vi "Set 1D Array String.vi"(5 "use temporary file? (F)":bool, 8 "error in":errorcluster, 9 "value":string[](array[string]), 10 "variable name":string, 11 "GOLPI ref. in":T1={"pipe handle"={"lv_proc.dll file path"=path "", "process instance handle"=[], "debug mode"=FALSE, "debug data"=[]}, "fast read timeout [ms]"=500, "fast read settle time [ms]"=10, "fast read to multiple [ms]"=1, "max elements per input line"=100, "slow read timeout [ms]"=5000, "stdin double format specifier"="%_16e", "max elements per stdout output column"=100, "console mode bitstream"=FALSE, "bitstream first read timeout [ms]"=1000, "bitstream read timeout [ms]"=50, "struct transfer possible"=FALSE, "matlab mode"=FALSE, "var pipe write timeout [ms]"=5000, "variable pipe mode"=FALSE, "variable pipe buffer size [Bytes]"=10000000, "variable pipe block size [Bytes]"=1000000} {"variable pipe block size [Bytes]" format="%.0p"; "variable pipe buffer size [Bytes]" format="%.0p"}) -> (0 "error out":errorcluster, 3 "GOLPI ref. out":T1={"pipe handle"={"lv_proc.dll file path"=path "", "process instance handle"=[], "debug mode"=FALSE, "debug data"=[]}, "fast read timeout [ms]"=500, "fast read settle time [ms]"=10, "fast read to multiple [ms]"=1, "max elements per input line"=100, "slow read timeout [ms]"=5000, "stdin double format specifier"="%_16e", "max elements per stdout output column"=100, "console mode bitstream"=FALSE, "bitstream first read timeout [ms]"=1000, "bitstream read timeout [ms]"=50, "struct transfer possible"=FALSE, "matlab mode"=FALSE, "var pipe write timeout [ms]"=5000, "variable pipe mode"=FALSE, "variable pipe buffer size [Bytes]"=10000000, "variable pipe block size [Bytes]"=1000000} {"variable pipe block size [Bytes]" format="%.0p"; "variable pipe buffer size [Bytes]" format="%.0p"})   [LabVIEW 2020, in "GOLPI library.lvlib"]
doc: "Part of polymorph Set Variable.vi"
uses:
  GOLPI library.lvlib
  Public/GOLPI reference Type Def.ctl
  LV Process source distribution/Pipe Handle.ctl
  LV Process source distribution/LV Process library.lvlib
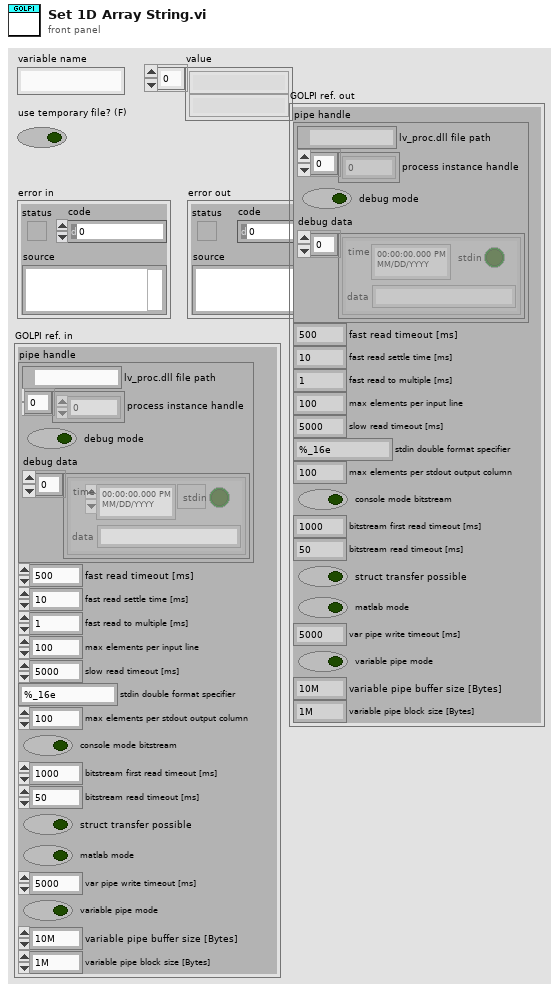
[diagram p1: front panel]
types:
  T1 = typedef "GOLPI library.lvlib/GOLPI reference Type Def.ctl" = cluster{"pipe handle":T2, "fast read timeout [ms]":u32, "fast read settle time [ms]":u32, "fast read to multiple [ms]":u32, "max elements per input line":u32, "slow read timeout [ms]":u32, "stdin double format specifier":string, "max elements per stdout output column":u32, "console mode bitstream":bool, "bitstream first read timeout [ms]":u32, "bitstream read timeout [ms]":u32, "struct transfer possible":bool, "matlab mode":bool, "var pipe write timeout [ms]":u32, "variable pipe mode":bool, "variable pipe buffer size [Bytes]":u32, "variable pipe block size [Bytes]":u32}
  T2 = typedef "LV Process library.lvlib/Pipe Handle.ctl" = cluster{"lv_proc.dll file path":path, "process instance handle":u32[], "debug mode":bool, "debug data":cluster{"time":timestamp, "stdin":bool, "data":string}[]}
  T3 = typedef "GOLPI library.lvlib/Transfer Mode.ctl" = enum16{"Matlab", "stdio", "temp file", "bitstream", "pipe"}
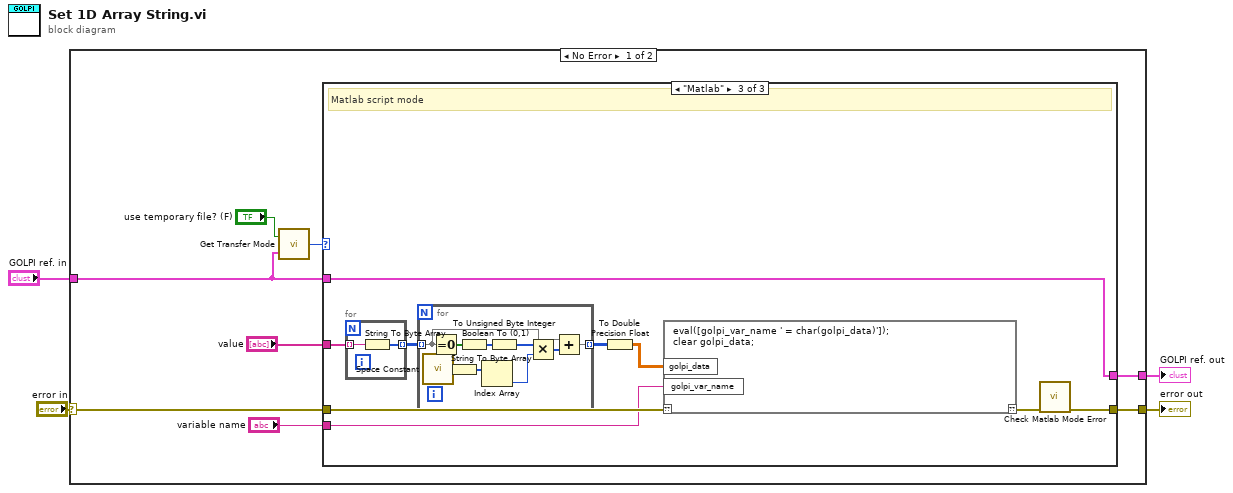
[diagram p0: block diagram]
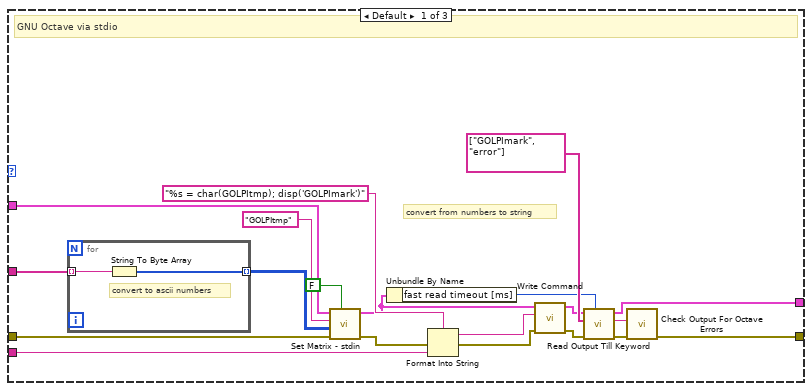
[diagram p2: hidden frame]
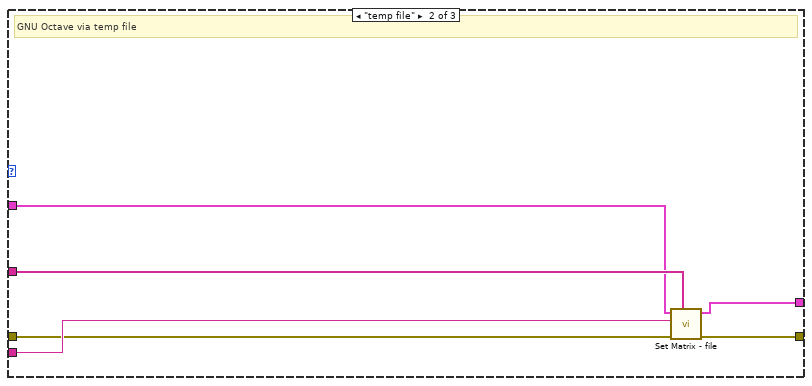
[diagram p3: hidden frame]
diagram:
  n1 = case shown="No Error" "error in" {
    selector: "error in" -> [w8 w62]
    tunnel: [w12 w62] -> w4
    tunnel: "GOLPI ref. in" -> [w6 w61]
    tunnel: [w11 w61] -> w1
    frame No Error {
      n2 = call "Get Transfer Mode.vi"("GOLPI ref."=w6, "use temporary file? (F)"="use temporary file? (F)") -> ("mode"=w7:T3)
      n3 = case shown="\"Matlab\"" w7 {
        tunnel: [w32 w40 w41] -> w12
        tunnel: [w31 w39 w43] -> w11
        tunnel: "variable name" -> [w30 w38 w48]
        tunnel: "value" -> [w29 w37 w47]
        tunnel: w8 -> [w28 w36 w49]
        tunnel: w6 -> [w27 w35 w43]
        frame Default {
          # "convert from numbers to string"
          # "GNU Octave via stdio"
          n4 = for {
            tunnel: w29 -> [w34] mode=indexing
            tunnel: [w33] -> w14 mode=indexing
            # "convert to ascii numbers"
            n5 = String To Byte Array(string=w34) -> (unsigned byte array=w33:u8[])
          }
          n6 = call "Set Matrix - stdin.vi"("swap dimensions? (F)"=FALSE ("swap dimensions?"), "error in"=w28, "value"=w14, "variable name"="GOLPItmp", "GOLPI ref. in"=w27) -> ("error out"=w16:errorcluster, "GOLPI ref. out"=w15:T1)  [unwired: 5 in]
          n7 = Unbundle By Name(w15) -> ("fast read timeout [ms]"=w18:u32)
          n8 = Format Into String(format string="%s = char(GOLPItmp); disp('GOLPImark')", error in=w16, w30) -> (resulting string=w24:string, error out=w25:errorcluster)  [unwired: 1 in]
          n9 = call "Write Command.vi"("error in"=w25, "command"=w24, "GOLPI ref. in"=w15) -> ("error out"=w23:errorcluster, "GOLPI ref. out"=w20:T1)  [unwired: 7 in]
          n10 = call "Read Output Till Keyword.vi"("timeout [ms]"=w18, "error in"=w23, "keywords"=string[] ["GOLPImark", "error"], "GOLPI ref. in"=w20) -> ("error out"=w22:errorcluster, "read buffer"=w19:string, "GOLPI ref. out"=w31:T1)  [unwired: 4 in, 1 out]
          n11 = call "Check Output For Octave Errors.vi"("error in"=w22, "read buffer"=w19) -> ("error out"=w32:errorcluster)  [unwired: 9 in]
        }
        frame "temp file" {
          # "GNU Octave via temp file"
          n12 = call "Set Matrix - file.vi"("string array"=w37, "error in (no error)"=w36, "variable name"=w38, "GOLPI ref. in"=w35) -> ("error out"=w40:errorcluster, "GOLPI ref. out"=w39:T1)  [unwired: 6 in]
        }
        frame "Matlab" {
          # "Matlab script mode"
          n13 = for {
            tunnel: w47 -> [w60] mode=indexing
            tunnel: [w59] -> w46 mode=indexing
            n14 = String To Byte Array(string=w60) -> (unsigned byte array=w59:u8[])
          }
          n15 = for {
            tunnel: w46 -> [w51] mode=indexing
            tunnel: [w50] -> w45 mode=indexing
            n16 = call <vilib>:"Space Constant.vi"() -> ("String"=w56:string)
            n17 = Equal To 0?(x=w51) -> (x = 0?=w58:bool[])
            n18 = String To Byte Array(string=w56) -> (unsigned byte array=w55:u8[])
            n19 = Boolean To (0,1)(Boolean=w58) -> (0, 1=w57:i16[])
            n20 = Index Array(array=w55) -> (element=w54:u8)  [unwired: 1 in]
            n21 = To Unsigned Byte Integer(number=w57) -> (unsigned 8bit integer=w53:u8[])
            n22 = Multiply(x=w53, y=w54) -> (x*y=w52:u8[])
            n23 = Add(x=w51, y=w52) -> (x+y=w50:u8[])
          }
          n24 = To Double Precision Float(number=w45) -> (double precision float=w44:dbl[][])
          n25 = script code="eval([golpi_var_name ' = char(golpi_data)']);\nclear golpi_data;"("??"=w49, "golpi_var_name"=w48, "golpi_data"=w44) -> ("??"=w42:errorcluster)
          n26 = call "Check Matlab Mode Error.vi"("error in"=w42) -> ("error out"=w41:errorcluster)  [unwired: 10 in]
        }
      }
    }
    frame Error {
    }
  }
  "error out" <- w4
  "GOLPI ref. out" <- w1
